vi "Digit value property.vi"(10 "Value":dbl, 11 "reference":refnum<vi>) -> ()   [LabVIEW 2022 SP3]
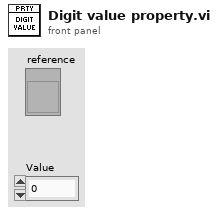
[diagram p1: front panel]
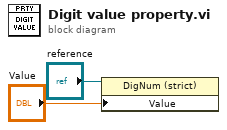
[diagram p0: block diagram]
diagram:
  n1 = property class="DigNum (strict)"(reference="reference", "Value"="Value") -> ()  [unwired: 1 in, 2 out]
